vi "Bot.vi"(7 "BotData":T4, 10 "MatchState":T1, 11 "GameState":T2) -> (0 "error out":errorcluster, 3 "Move":T5)   [LabVIEW 2015, in "ReplayBot.lvlib"]
uses:
  ReplayBot.lvlib
  TronVIEWBotAPI/MovementDirection.ctl
  TronVIEWBotAPI/BotData.ctl
  TronVIEWBotAPI/GameState.ctl
  TronviewGame/Board/Position.ctl
  TronVIEWBotAPI/MatchState.ctl
  TronVIEWBotAPI/TronVIEWBotAPI.lvlib
  TronviewGame/Board/Board.lvclass
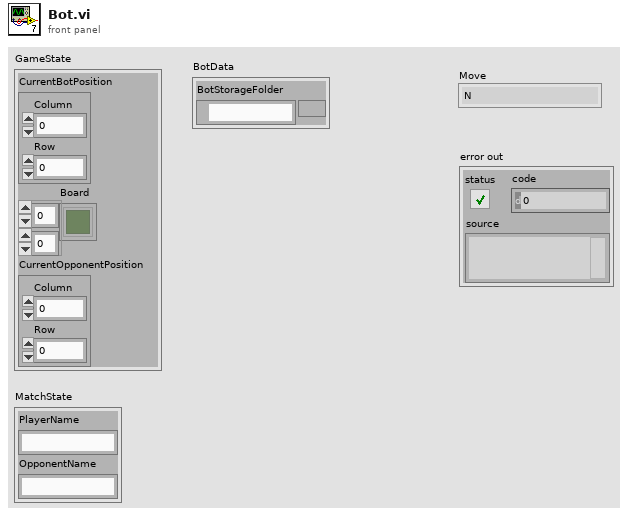
[diagram p1: front panel]
types:
  T1 = typedef "TronVIEWBotAPI.lvlib/MatchState.ctl" = cluster{"PlayerName":string, "OpponentName":string}
  T2 = typedef "TronVIEWBotAPI.lvlib/GameState.ctl" = cluster{"CurrentBotPosition":T3, "Board":bool[][], "CurrentOpponentPosition":T3}
  T3 = typedef "TronviewGame.lvlib/Board.lvclass/Position.ctl" = cluster{"Column":i32, "Row":i32}
  T4 = typedef "TronVIEWBotAPI.lvlib/BotData.ctl" = cluster{"BotStorageFolder":path}
  T5 = typedef "TronVIEWBotAPI.lvlib/MovementDirection.ctl" = enum16{"N", "S", "W", "E"}
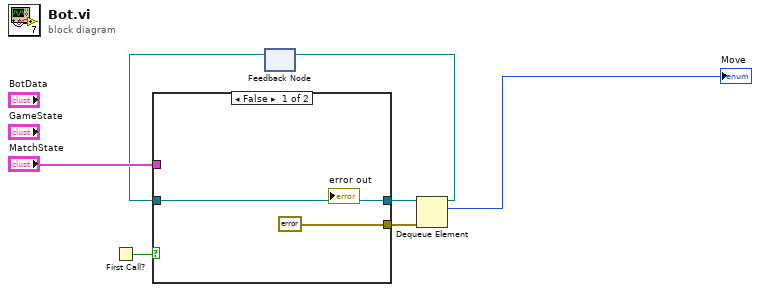
[diagram p0: block diagram]
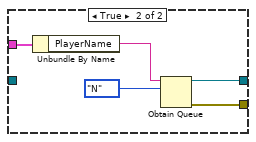
[diagram p2: hidden frame]
diagram:
  n1 = First Call?() -> (First Call?: T/F=w6:bool)
  n2 = feedback #1() -> (w1:refnum<queue>)  [unwired: 1 in]
  n3 = case shown="False" w6 {
    tunnel: "MatchState" -> [_ w14]
    tunnel: [w9 w11] -> w5
    tunnel: [errorcluster {"status"=FALSE, "code"=0, "source"=""} ("error out") w10] -> w4
    tunnel: w1 -> [w9 _]
    frame False {
    }
    frame True {
      n4 = Unbundle By Name(w14) -> ("PlayerName"=w13:string)
      n5 = Obtain Queue(name (unnamed)=w13, element data type=MovementDirection."N" ("Direction")) -> (queue out=w11:refnum<queue>, error out=w10:errorcluster)  [unwired: 3 in, 1 out]
    }
  }
  n6 = Dequeue Element(queue=w5, error in (no error)=w4) -> (queue out=w2:refnum<queue>, element=→"Move":T5)  [unwired: 1 in, 2 out]
  n7 = feedback-in #1(w2) -> ()
